vi "Ew.vi"(1 "Measured Drag Coeff. (Cdm)":dbl, 2 "Vehicle Frontal Area (Am)":dbl, 3 "Collector Area (Ac)":dbl) -> (0 "Wake Blockage Factor (Ew)":dbl)   [LabVIEW 2017]
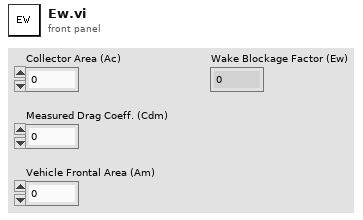
[diagram p1: front panel]
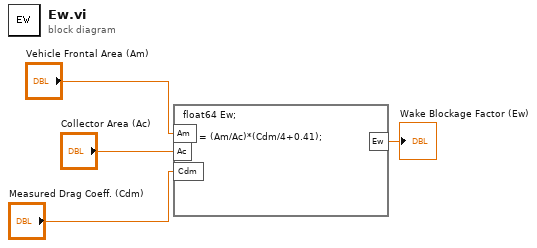
[diagram p0: block diagram]
diagram:
  n1 = formula code="float64 Ew;\n\nEw = (Am/Ac)*(Cdm/4+0.41);"("Am"="Vehicle Frontal Area (Am)", "Ac"="Collector Area (Ac)", "Cdm"="Measured Drag Coeff. (Cdm)") -> ("Ew"=→"Wake Blockage Factor (Ew)":dbl)
